vi "FindPath.vi"(9 "Wall Angle (Relative)":dbl, 10 "Lidar Angles":dbl[](array[numeric]), 11 "Lidar Distances":dbl[](array[numeric])) -> (3 "Direction to move in (deg)":dbl)   [LabVIEW 2016]
uses:
  <vilib>/robotics/Obstacle Avoidance/Advanced Vector Field Histogram/NI_Robotics_Vector Field Histogram.lvlib
panel:
  out "error out":errorcluster
  out "Waveform Chart":dbl[](graph)
  out "LIDAR Data and Path":cluster{dbl[], dbl[]}(graph)
  # "Given the LIDAR data, return a direction which we can move in to get past the obstacles."
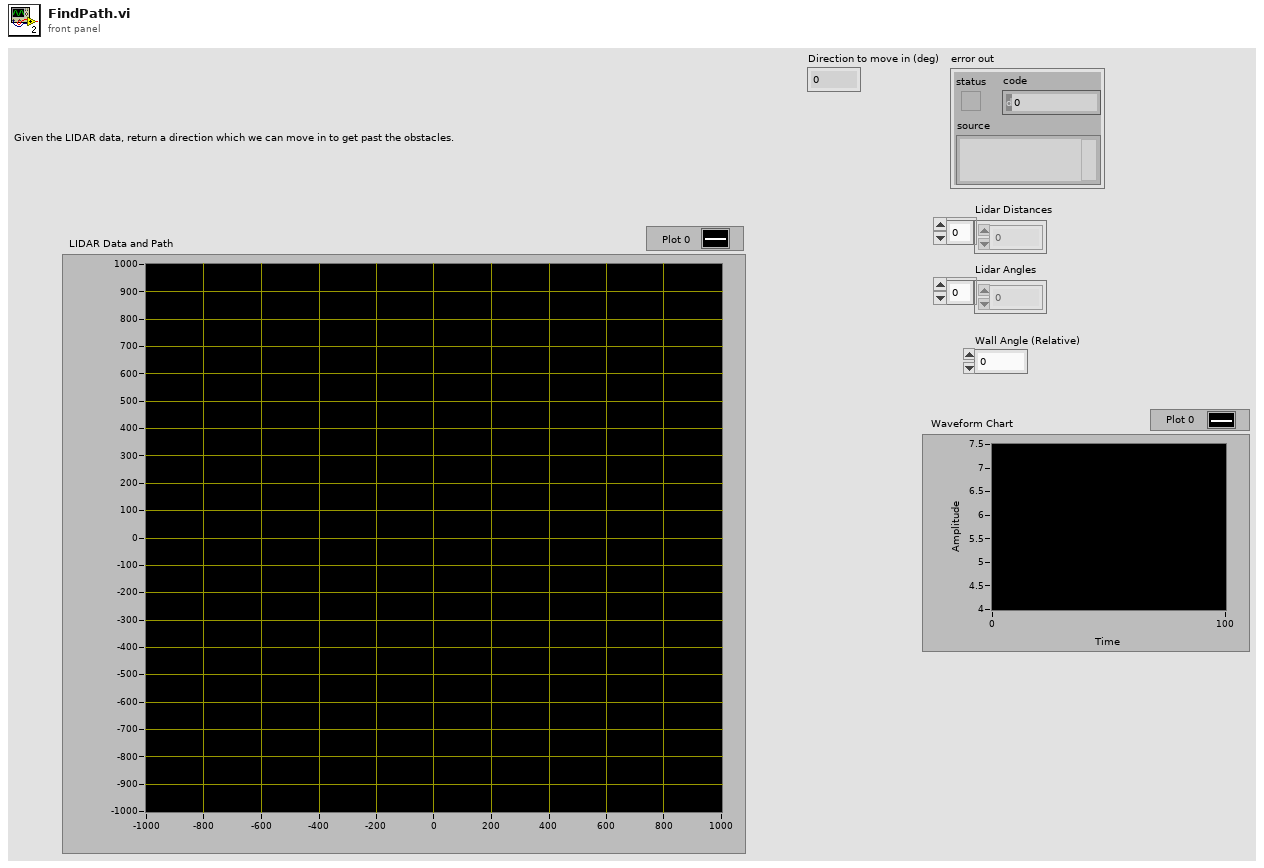
[diagram p1: front panel]
types:
  T1 = cluster{"inner threshold distance":dbl, "outer threshold distance":dbl}
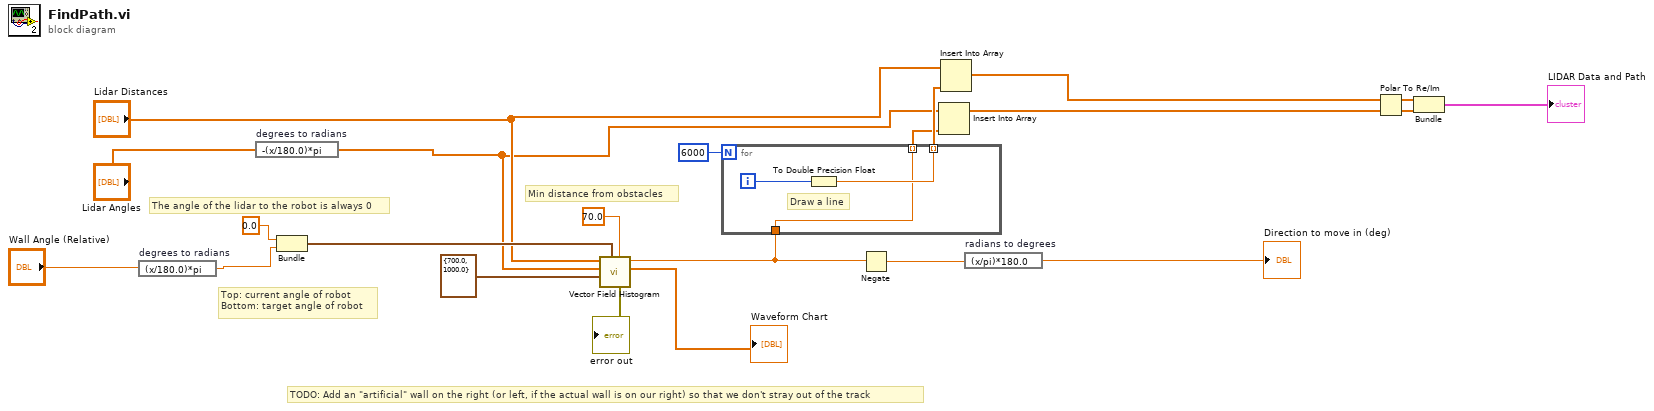
[diagram p0: block diagram]
diagram:
  # "TODO: Add an \"artificial\" wall on the right (or left, if the actual wall is on our right) so that we don't stray out of the track"
  # "The angle of the lidar to the robot is always 0"
  # "Top: current angle of robot\nBottom: target angle of robot"
  # "Min distance from obstacles"
  n1 = expression code="(x/180.0)*pi" "degrees to radians"("Wall Angle (Relative)") -> (w10:dbl)
  n2 = expression code="-(x/180.0)*pi" "degrees to radians"("Lidar Angles") -> (w6:dbl[])
  n3 = Bundle(0.0, "Wall Angle (Relative)"=w10) -> (w18:cluster{dbl, "Wall Angle (Relative)":dbl})  [unwired: 1 in]
  n4 = call <vilib>:"Vector Field Histogram.vi"("obstacle clearance distance"=70.0, "heading"=w18, "thresholds"=T1 {"inner threshold distance"=700.0, "outer threshold distance"=1000.0}, "direction angles (rad)"=w6, "distances"="Lidar Distances") -> ("error out"=→"error out":errorcluster, "histogram"=→"Waveform Chart":dbl[], "chosen heading (rad)"=w2:dbl)  [unwired: 3 in, 1 out]
  n5 = for {
    N: 6000 -> [_]
    tunnel: w2 -> [w23]
    tunnel: [w24] -> w12 mode=indexing
    tunnel: [w23] -> w11 mode=indexing
    i -> [w25]
    # "Draw a line"
    n6 = To Double Precision Float(number=w25) -> (double precision float=w24:dbl)
  }
  n7 = Negate(x=w2) -> (-x=w1:dbl)
  n8 = Insert Into Array(array=w6, new element=w11) -> (w8:dbl[])  [unwired: 1 in]
  n9 = Insert Into Array(array="Lidar Distances", new element=w12) -> (w9:dbl[])  [unwired: 1 in]
  n10 = expression code="(x/pi)*180.0" "radians to degrees"(w1) -> (→"Direction to move in (deg)":dbl)
  n11 = Polar To Re/Im(2:w8, 3:w9) -> (0:w14:dbl[], 1:w15:dbl[])
  n12 = Bundle(w15, w14) -> (→"LIDAR Data and Path":cluster{dbl[], dbl[]})  [unwired: 1 in]
